vi "TonesLoop_20190705.vi"(7 "WeightOfNewFrequency":dbl=0.1 format="%#_13g", 8 "error in":errorcluster, 11 "Queue in":refnum<queue>) -> (0 "error out":errorcluster)   [LabVIEW 2018]
uses:
  Queue/DataQueueElements.ctl
  Controls/Clusts/ChannelToneData.ctl
  Controls/ToneInfoClust.ctl
  Controls/Clusts/TargetToneData.ctl
  Controls/Clusts/SaturationMonitor.ctl
  Controls/Clusts/Tones_Loop.ctl
  Controls/Clusts/Config_Clust.ctl
  Controls/Clusts/UserConfig.ctl
  Controls/PathsCluster.ctl
  Controls/Clusts/FrontPanel_UserConfig.ctl
  Controls/Clusts/Inclinometer_User_Cfg.ctl
  Controls/Clusts/FP_UserTargetConfig.ctl
  Controls/Clusts/FreqShift.ctl
  Controls/Clusts/FPGA_Scale.ctl
  Controls/Enums/ScaleMeasure.ctl
  Controls/RadioButtons/FilterEnableRadio.ctl
  Controls/Enums/TargetNumber.ctl
  Controls/Clusts/FPGA_Config_Clust.ctl
  Controls/Clusts/NowAllTones.ctl
  Controls/Clusts/FreqFilePaths.ctl
  Controls/Clusts/TonesLogAll.ctl
  Controls/Clusts/ToneLogBuffered.ctl
  Controls/Clusts/SaturationMonitorBuffer.ctl
  Controls/Clusts/AcqData.ctl
  Controls/Clusts/FromFPGA_Clust.ctl
  Controls/Enums/LogLoopEnum.ctl
  Controls/Enums/FP_Loop_Enum.ctl
  Controls/Enums/WatchdogTimer_Enum.ctl
  Controls/Enums/10Hz_Loop_Enum.ctl
  Controls/Clusts/10Hz_Data.ctl
panel:
  in  "1":T1={"Cal"={"Shift_"=-24999462.633451957, "Peak_ToFPGA"=-24999462.633451957, "MaxValue"=0.0, "MaxIndex"=0, "Tone"={"PkLocTrak"=0.0, "PkLocDisp"=0.0, "df_"=0.0, "ZoomPwr"=[], "Phase"=0.0, "PhaseOld"=0.0, "AboveThresh?"=FALSE, "MaxI"=0.0, "MaxQ"=0.0, "median"=0.0, "ISpect"=[], "QSpect"=[], "DeltaPhase"=0.0}, "TimeDomainI"=array[12500 elements], "TimeDomainQ"=array[12500 elements], "PwrSpectrum"=[], "RunningAvgFreq"=0.0, "ISpectPos"=[], "ISpectNeg"=[], "QSpectPos"=[], "QSpectNeg"=[], "10Hz_PwrSpectr"=[], "SNR"=0.0, "AliasWarn"=FALSE, "10Hz_Peak"=[], "ISpect+-"=[], "QSpect+-"=[], "TimeStamp"=timestamp(0 s since 1904-01-01), "I_Index"=array[12500 elements], "Q_Index"=array[12500 elements], "10MHz"=FALSE}, "Beac"={"Shift_"=-24999462.633451957, "Peak_ToFPGA"=-24999462.633451957, "MaxValue"=0.0, "MaxIndex"=0, "Tone"={"PkLocTrak"=0.0, "PkLocDisp"=0.0, "df_"=0.0, "ZoomPwr"=[], "Phase"=0.0, "PhaseOld"=0.0, "AboveThresh?"=FALSE, "MaxI"=0.0, "MaxQ"=0.0, "median"=0.0, "ISpect"=[], "QSpect"=[], "DeltaPhase"=0.0}, "TimeDomainI"=array[12500 elements], "TimeDomainQ"=array[12500 elements], "PwrSpectrum"=[], "RunningAvgFreq"=0.0, "ISpectPos"=[], "ISpectNeg"=[], "QSpectPos"=[], "QSpectNeg"=[], "10Hz_PwrSpectr"=[], "SNR"=0.0, "AliasWarn"=FALSE, "10Hz_Peak"=[], "ISpect+-"=[], "QSpect+-"=[], "TimeStamp"=timestamp(0 s since 1904-01-01), "I_Index"=array[12500 elements], "Q_Index"=array[12500 elements], "10MHz"=FALSE}, "Time"=[], "Saturat"={"MeasMean0"=0.0, "MeasMean1"=0.0, "MeasMax"=0.0, "1_Max"=0.0, "4_Max"=0.0, "5_Max"=0.0, "6_Max"=0.0, "7_Max"=0.0}} {"Beac"."Tone"."median" format="%0.2f"; "Beac"."Tone"."MaxQ" format="%0.2f"; "Cal"."Tone"."median" format="%0.2f"; "Cal"."Tone"."MaxQ" format="%0.2f"}
  in  "Cal":T2={"Shift_"=-24999462.633451957, "Peak_ToFPGA"=-24999462.633451957, "MaxValue"=0.0, "MaxIndex"=0, "Tone"={"PkLocTrak"=0.0, "PkLocDisp"=0.0, "df_"=0.0, "ZoomPwr"=[], "Phase"=0.0, "PhaseOld"=0.0, "AboveThresh?"=FALSE, "MaxI"=0.0, "MaxQ"=0.0, "median"=0.0, "ISpect"=[], "QSpect"=[], "DeltaPhase"=0.0}, "TimeDomainI"=array[12500 elements], "TimeDomainQ"=array[12500 elements], "PwrSpectrum"=[], "RunningAvgFreq"=0.0, "ISpectPos"=[], "ISpectNeg"=[], "QSpectPos"=[], "QSpectNeg"=[], "10Hz_PwrSpectr"=[], "SNR"=0.0, "AliasWarn"=FALSE, "10Hz_Peak"=[], "ISpect+-"=[], "QSpect+-"=[], "TimeStamp"=timestamp(0 s since 1904-01-01), "I_Index"=array[12500 elements], "Q_Index"=array[12500 elements], "10MHz"=FALSE} {"Tone"."median" format="%0.2f"; "Tone"."MaxQ" format="%0.2f"}
  in  "CrossNew":bool
  in  "CoNew":bool
  out "Discard 4":i32
  out "Discard 3":i32
  out "Discard 2":i32
  out "Discard 1":i32
  out "Discard":i32
  out "4 Shift":i32
  out "3 Shift":i32
  out "2 Shift":i32
  out "1 Shift":i32
  out "4 Send":i32
  out "3 Send":i32
  out "2 Send":i32
  out "1 Send":i32
  out "4 Count":i32
  out "3 Count":i32
  out "2 Count":i32
  out "1Count":i32
  out "Tones_Count":i32
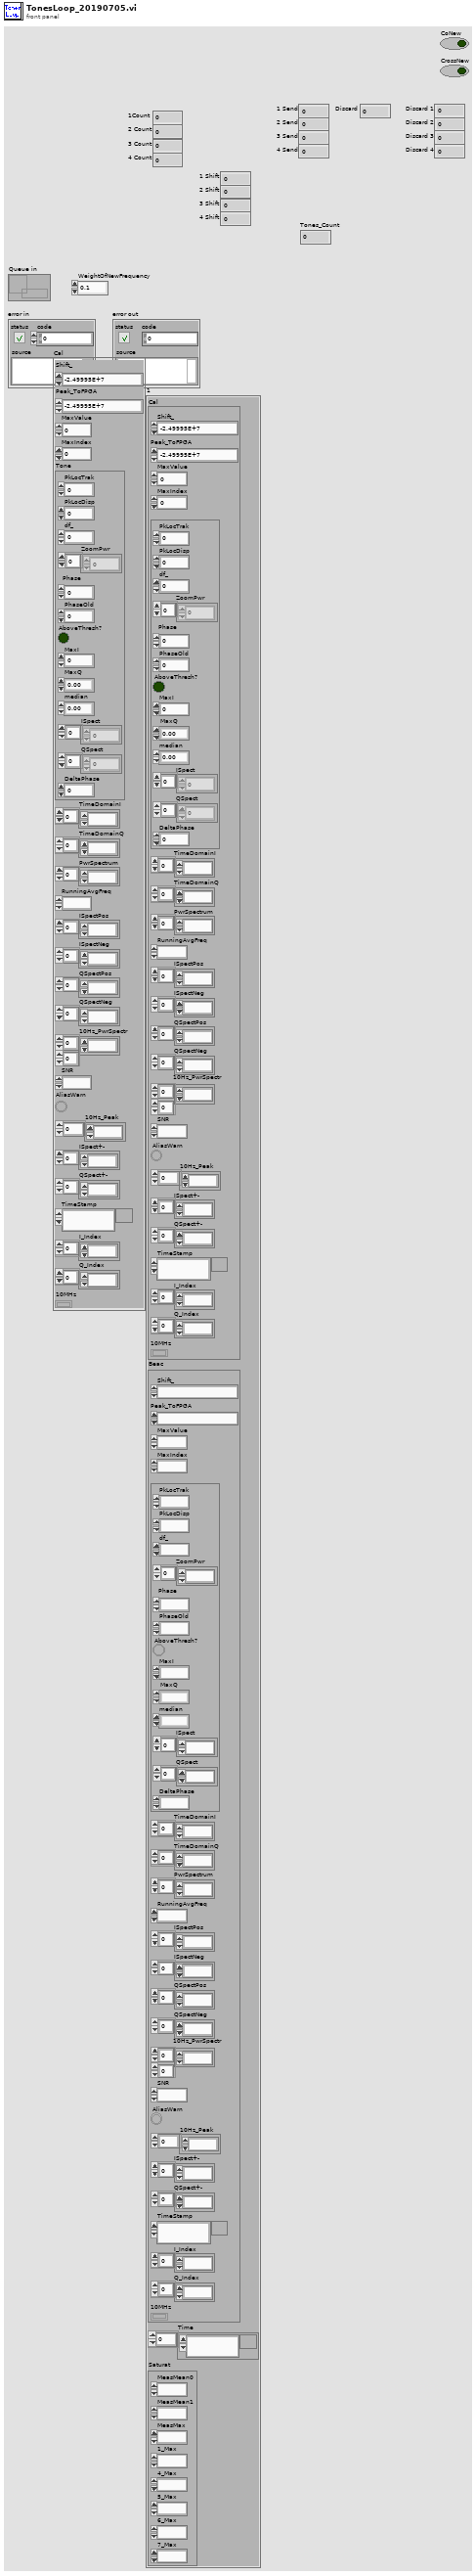
[diagram p1: front panel]
types:
  T1 = typedef "TargetToneData.ctl" = cluster{"Cal":T2, "Beac":T2, "Time":timestamp[], "Saturat":T4}
  T2 = typedef "ChannelToneData.ctl" = cluster{"Shift_":dbl, "Peak_ToFPGA":dbl, "MaxValue":dbl, "MaxIndex":i32, "Tone":T3, "TimeDomainI":ext[], "TimeDomainQ":ext[], "PwrSpectrum":dbl[], "RunningAvgFreq":dbl, "ISpectPos":dbl[], "ISpectNeg":dbl[], "QSpectPos":dbl[], "QSpectNeg":dbl[], "10Hz_PwrSpectr":dbl[][], "SNR":dbl, "AliasWarn":bool, "10Hz_Peak":dbl[], "ISpect+-":dbl[], "QSpect+-":dbl[], "TimeStamp":timestamp, "I_Index":ext[], "Q_Index":ext[], "10MHz":bool}
  T3 = typedef "ToneInfoClust.ctl" = cluster{"PkLocTrak":dbl, "PkLocDisp":dbl, "df_":dbl, "ZoomPwr":dbl[], "Phase":dbl, "PhaseOld":dbl, "AboveThresh?":bool, "MaxI":dbl, "MaxQ":dbl, "median":dbl, "ISpect":dbl[], "QSpect":dbl[], "DeltaPhase":dbl}
  T4 = typedef "SaturationMonitor.ctl" = cluster{"MeasMean0":dbl, "MeasMean1":dbl, "MeasMax":dbl, "1_Max":dbl, "4_Max":dbl, "5_Max":dbl, "6_Max":dbl, "7_Max":dbl}
  T5 = typedef "TonesLogAll.ctl" = cluster{"72co":T6, "72x":T6, "84co":T6, "84x":T6}
  T6 = typedef "ToneLogBuffered.ctl" = cluster{"Count":i32, "CalVal":sgl[], "CalLoc":i32[], "BeacVal":sgl[], "BeacLoc":i32[], "BeacShift":i32[], "Enum":T7, "df":dbl, "PwrSpectr":sgl[][], "ISpectr":sgl[][], "QSpectr":sgl[][], "Time":timestamp[], "SNR":sgl[], "AboveThresh":bool[], "10Hz_PeakVal":dbl[], "Phase":sgl[], "DeltaPhase":dbl[], "Saturat":T8, "10MHz":bool}
  T7 = typedef "TargetNumber.ctl" = enum16{"1", "2", "3", "4"}
  T8 = typedef "SaturationMonitorBuffer.ctl" = cluster{"Meas":bool[], "Stage1":bool[], "Stage4":bool[], "Stage5":bool[], "Stage6":bool[], "Stage7":bool[]}
  T9 = typedef "Tones_Loop.ctl" = cluster{"Config":T10, "FPGA":T20, "Now":T21, "FreqFiles":T22}
  T10 = typedef "Config_Clust.ctl" = cluster{"UsrCfg":T11, "FP_User":T13}
  T11 = typedef "UserConfig.ctl" = cluster{"Paths":T12, "SampleRate":dbl}
  T12 = typedef "PathsCluster.ctl" = cluster{"CfgFile":path, "LogFolder":path, "LogFile":path, "NAS path":path, "ThreshFile":path, "RedunFolder":path}
  T13 = typedef "FrontPanel_UserConfig.ctl" = cluster{"#NoiseSums":u32, "Max_df":u32, "AvgAvg":bool, "#Avg":u16, "AutoCenter":bool, "Inclin":T14, "1":T15, "2":T15, "3":T15, "4":T15, "Target to Probe":T7, "SNR_Thresh":dbl, "Paths":T12, "Connex_Location":string, "SimulateFPGA":bool, "Deadband":dbl}
  T14 = typedef "Inclinometer_User_Cfg.ctl" = cluster{"Vmin":dbl, "Vmax":dbl, "Angle_min":dbl, "Angle_max":dbl, "Offset":dbl, "Pos_Neg":bool}
  T15 = typedef "FP_UserTargetConfig.ctl" = cluster{"Cal_":T16, "Beac":T16, "Scale":T17, "Offset":fxp<+/-,16,16>, "Scale_Noise":fxp<+/-,30,30>, "Scale_Step1":fxp<+/-,17,17>, "Scale_In_RT":ext, "ScaleMeas":fxp<+/-,16,1>, "FreqsToRemove":i32[], "Width":i32[], "ScaleMeasEnum":T18, "FilterEnab":T19}
  T16 = typedef "FreqShift.ctl" = cluster{"Fine":dbl, "Coarse_":dbl}
  T17 = typedef "FPGA_Scale.ctl" = cluster{"Step4":fxp<+/-,23,23>, "Step5":fxp<+/-,23,23>, "Step6":fxp<+/-,23,23>, "Step7":fxp<+/-,23,23>}
  T18 = typedef "ScaleMeasure.ctl" = enum16{"1", "10", "50", "42"}
  T19 = typedef "FilterEnableRadio.ctl" = enum32{"None", "Step 1", "Frequency Shift", "Step 4", "Step 5", "Step 6", "Step 7"}
  T20 = typedef "FPGA_Config_Clust.ctl" = cluster{"Target":T7, "Channel":T7, "Ref1":refnum<k20>, "Ref2":refnum<k20>}
  T21 = typedef "NowAllTones.ctl" = cluster{"Target":T7, "SampleRate":dbl, "AvgFreq":dbl, "72_Shift_":dbl, "84_Shift_":dbl, "1":T1, "2":T1, "3":T1, "4":T1}
  T22 = typedef "FreqFilePaths.ctl" = cluster{"72":path, "84":path}
  T23 = typedef "AcqData.ctl" = cluster{"Data":fxp<+/-,24,1>[], "#":T7, "Saturat":T4, "FromFPGA":T24, "10MHz":bool}
  T24 = typedef "FromFPGA_Clust.ctl" = cluster{"CalTimeDomainI":ext[], "CalTimeDomainI.Index":ext[], "CalTimeDomainQ":ext[], "CalTimeDomainQ.Index":ext[], "BeacTimeDomainI":ext[], "BeacTimeDomainI.Index":ext[], "BeacTimeDomainQ":ext[], "BeacTimeDomainQ.Index":ext[]}
  T25 = typedef "WatchdogTimer_Enum.ctl" = enum16{"ResetAll", "CheckAll", "HW1", "HW2", "Tones", "FP", "Noise", "Log", "TCP", "AI", "TC", "ADAM", "Disdrom", "TE", "Weather"}
  T26 = typedef "FP_Loop_Enum.ctl" = enum16{"FP_Init", "FP_Scale", "FP_Tone", "FP_Noise", "FP_Probes", "FP_PXI", "FP_AI", "FP_TC", "FP_PWR_Hist", "FP_Alarm", "FP_Exit"}
  T27 = typedef "LogLoopEnum.ctl" = enum16{"Log_Init", "Log_Config", "Log_CfgAlarm", "Log_TimeDomain", "Log_Tone", "Log_NoiseTrace", "Log_NoiseSum", "Log_DO", "Log_AI", "Log_TC", "Log_Disdrom", "Log_Weather", "Log_TE", "Log_ADAM", "Log_UPS", "Log_ChkTime", "Log_Alarm", "Log_SSH", "Log_Write", "Log_Exit"}
  T28 = typedef "10Hz_Data.ctl" = cluster{"PeakVal":dbl[], "Channel":T7, "TimeStamp":timestamp}
  T29 = typedef "10Hz_Loop_Enum.ctl" = enum16{"10Hz_Init", "10Hz_Cfg", "10Hz_NewData", "10Hz_Write", "10Hz_Stop"}
  T30 = typedef "DataQueueElements.ctl" = enum16{"Data_Init", "Data_Config", "Data_AddData", "Data_FreqShift", "Data_FPGA_Write", "Data_Transform", "Data_Send", "Data_Exit"}
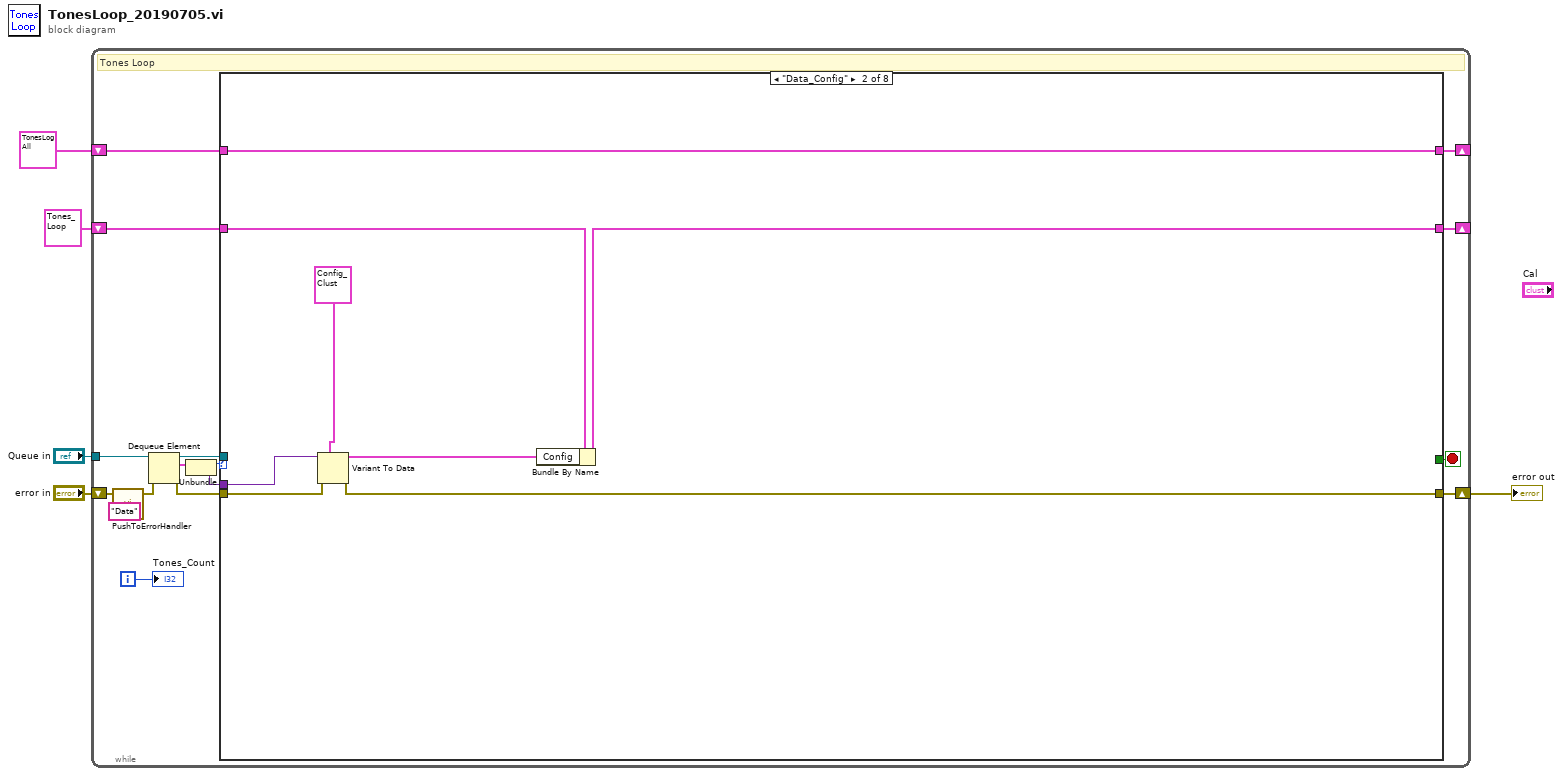
[diagram p0: block diagram]
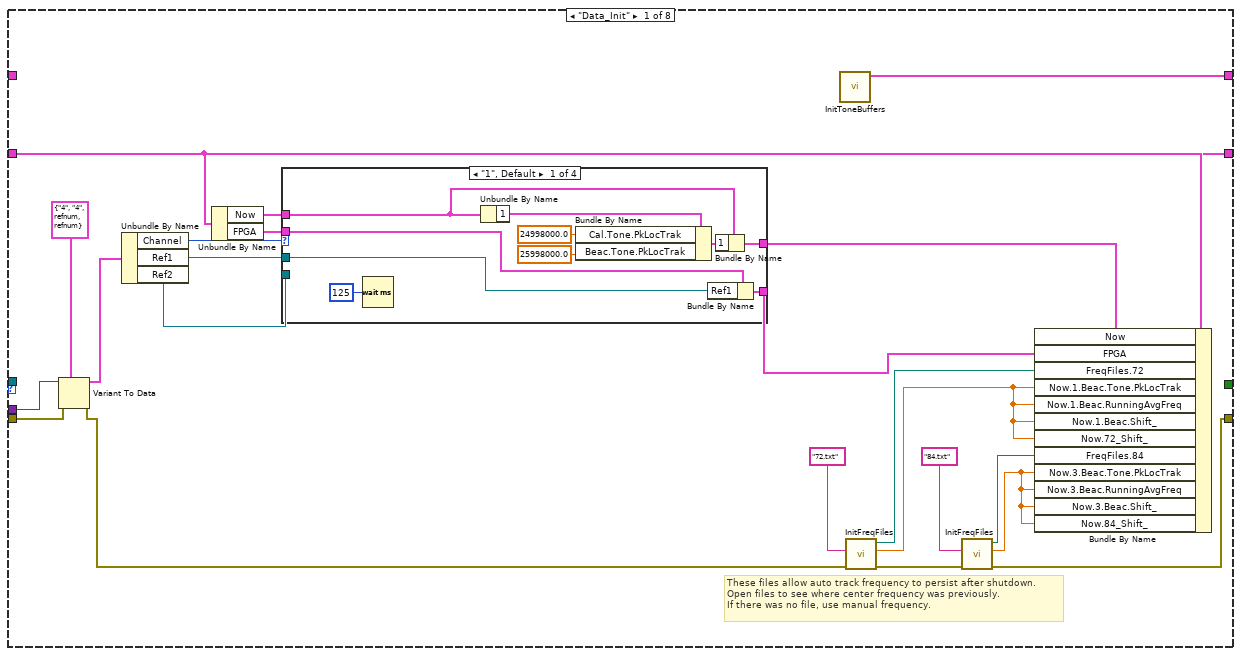
[diagram p2: hidden frame]
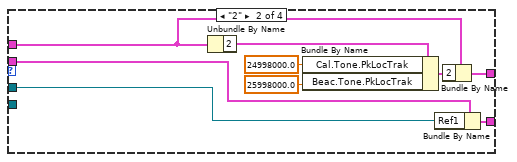
[diagram p3: hidden frame]
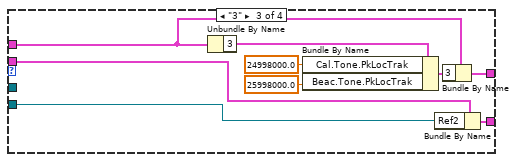
[diagram p4: hidden frame]
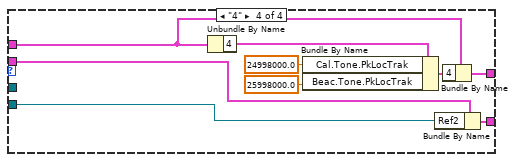
[diagram p5: hidden frame]
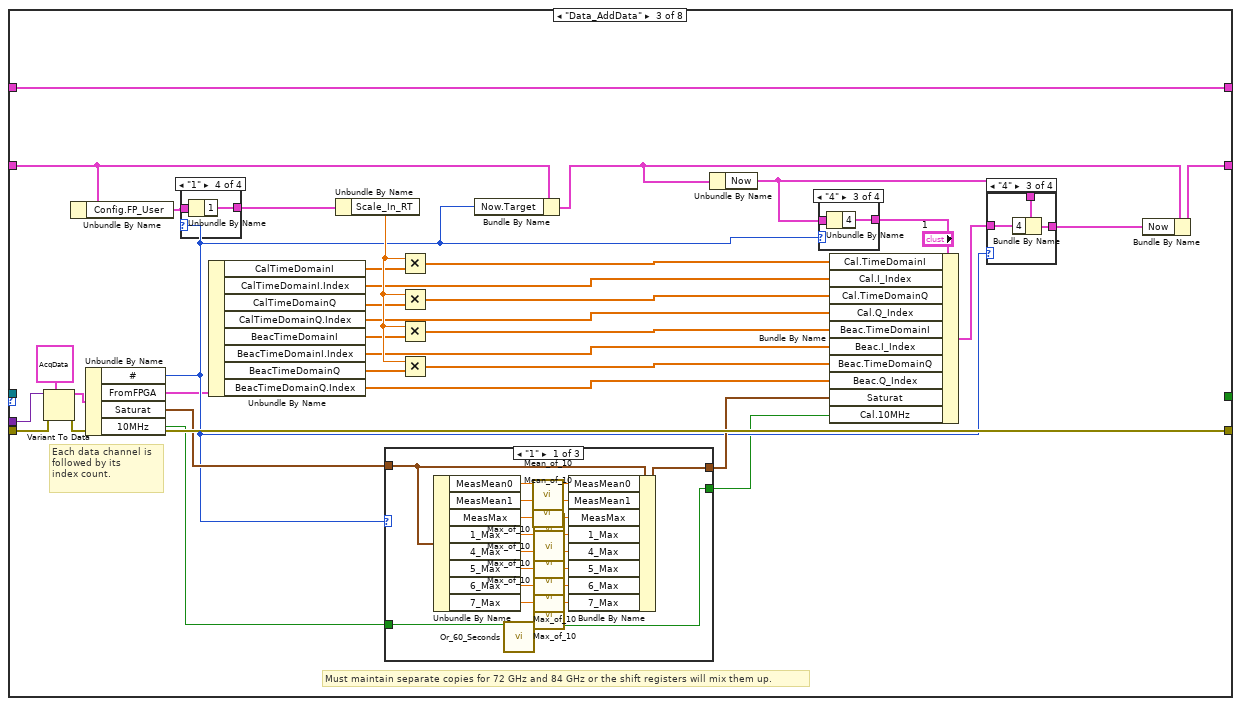
[diagram p6: hidden frame]
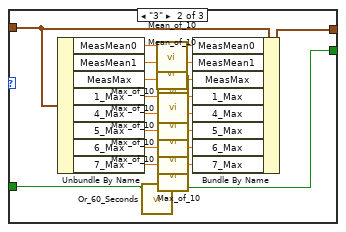
[diagram p7: hidden frame]
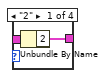
[diagram p9: hidden frame]
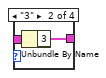
[diagram p10: hidden frame]
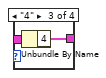
[diagram p11: hidden frame]
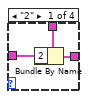
[diagram p12: hidden frame]
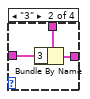
[diagram p13: hidden frame]
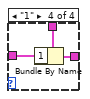
[diagram p14: hidden frame]
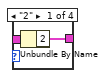
[diagram p15: hidden frame]
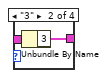
[diagram p16: hidden frame]
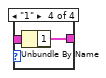
[diagram p17: hidden frame]
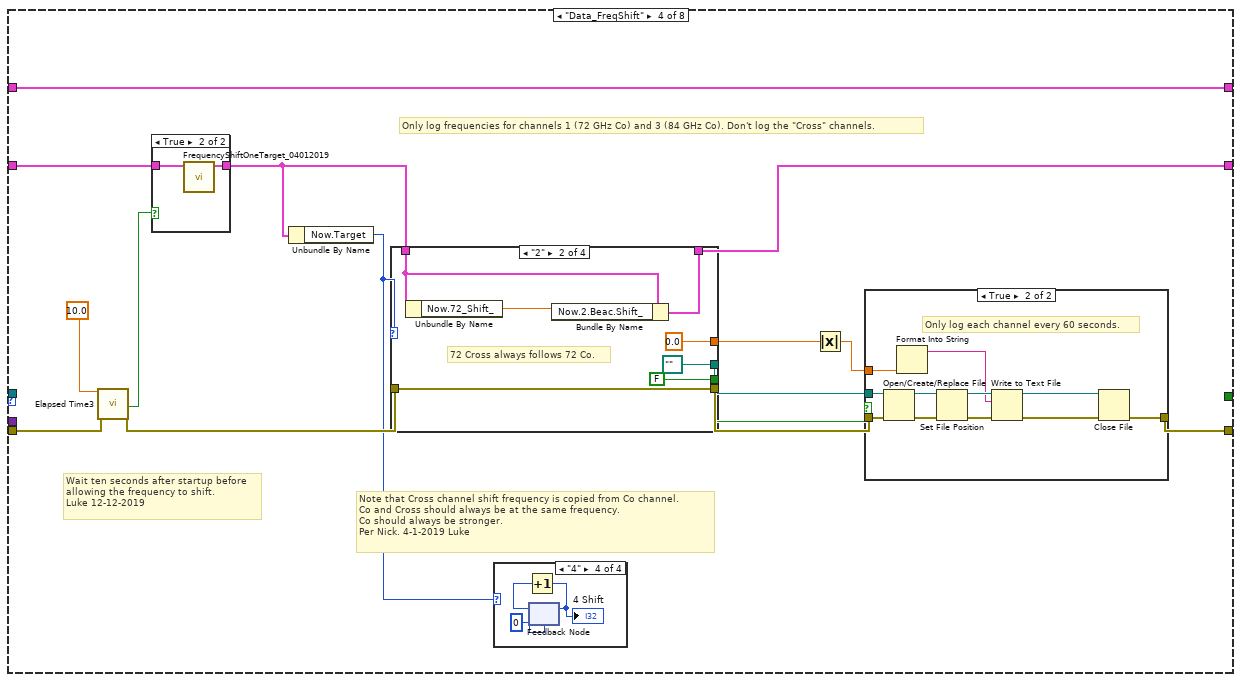
[diagram p18: hidden frame]
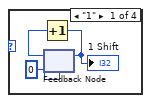
[diagram p19: hidden frame]
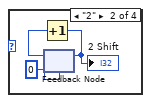
[diagram p20: hidden frame]
diagram:
  n1 = while {
    shift-right: [w14] -> w3
    shift-left: "error in" -> [w19]
    tunnel: "Queue in" -> [w7]
    shift-right: [w11] -> _
    shift-left: T9 {"Config"={"UsrCfg"={"Paths"={"CfgFile"=path "", "LogFolder"=path "", "LogFile"=path "", "NAS path"=path "", "ThreshFile"=path "", "RedunFolder"=path ""}, "SampleRate"=12500.0}, "FP_User"={"#NoiseSums"=1, "Max_df"=1, "AvgAvg"=FALSE, "#Avg"=1, "AutoCenter"=FALSE, "Inclin"={"Vmin"=0.0, "Vmax"=0.0, "Angle_min"=0.0, "Angle_max"=0.0, "Offset"=0.0, "Pos_Neg"=FALSE}, "1"={"Cal_"={"Fine"=0.000213623046875, "Coarse_"=4194303.0}, "Beac"={"Fine"=4194303.0, "Coarse_"=1.0}, "Scale"={"Step4"=10000.0, "Step5"=4194303.0, "Step6"=1.0, "Step7"=10000.0}, "Offset"=0.0, "Scale_Noise"=4194303.0, "Scale_Step1"=65535.0, "Scale_In_RT"=1.0, "ScaleMeas"=0.999969482421875, "FreqsToRemove"=[0, 1633], "Width"=[0, 1633], "ScaleMeasEnum"=enum."50", "FilterEnab"=enum."Step 1"}, "2"={"Cal_"={"Fine"=0.000213623046875, "Coarse_"=4194303.0}, "Beac"={"Fine"=0.000213623046875, "Coarse_"=4194303.0}, "Scale"={"Step4"=0.0, "Step5"=4194303.0, "Step6"=1.0, "Step7"=10000.0}, "Offset"=0.0, "Scale_Noise"=4194303.0, "Scale_Step1"=65535.0, "Scale_In_RT"=1.0, "ScaleMeas"=0.999969482421875, "FreqsToRemove"=[0, 1633], "Width"=[0, 1633], "ScaleMeasEnum"=enum."50", "FilterEnab"=enum."Step 1"}, "3"={"Cal_"={"Fine"=0.000213623046875, "Coarse_"=4194303.0}, "Beac"={"Fine"=0.000213623046875, "Coarse_"=4194303.0}, "Scale"={"Step4"=0.0, "Step5"=4194303.0, "Step6"=1.0, "Step7"=10000.0}, "Offset"=0.0, "Scale_Noise"=4194303.0, "Scale_Step1"=65535.0, "Scale_In_RT"=1.0, "ScaleMeas"=0.999969482421875, "FreqsToRemove"=[0, 1633], "Width"=[0, 1633], "ScaleMeasEnum"=enum."50", "FilterEnab"=enum."Step 1"}, "4"={"Cal_"={"Fine"=0.000213623046875, "Coarse_"=4194303.0}, "Beac"={"Fine"=0.000213623046875, "Coarse_"=4194303.0}, "Scale"={"Step4"=0.0, "Step5"=4194303.0, "Step6"=1.0, "Step7"=10000.0}, "Offset"=0.0, "Scale_Noise"=4194303.0, "Scale_Step1"=1.0, "Scale_In_RT"=10000.0, "ScaleMeas"=0.999969482421875, "FreqsToRemove"=[0, 1633], "Width"=[0, 1633], "ScaleMeasEnum"=enum."50", "FilterEnab"=enum."Step 1"}, "Target to Probe"=enum."4", "SNR_Thresh"=1.0, "Paths"={"CfgFile"=path "", "LogFolder"=path "", "LogFile"=path "", "NAS path"=path "", "ThreshFile"=path "", "RedunFolder"=path ""}, "Connex_Location"="", "SimulateFPGA"=FALSE, "Deadband"=0.0}}, "FPGA"={"Target"=enum."4", "Channel"=enum."4", "Ref1"=refnum, "Ref2"=refnum}, "Now"={"Target"=enum."4", "SampleRate"=0.0, "AvgFreq"=0.0, "72_Shift_"=-24999462.633451957, "84_Shift_"=-24999462.633451957, "1"={"Cal"={"Shift_"=-24999462.633451957, "Peak_ToFPGA"=-24999462.633451957, "MaxValue"=0.0, "MaxIndex"=0, "Tone"={"PkLocTrak"=0.0, "PkLocDisp"=0.0, "df_"=0.0, "ZoomPwr"=[], "Phase"=0.0, "PhaseOld"=0.0, "AboveThresh?"=FALSE, "MaxI"=0.0, "MaxQ"=0.0, "median"=0.0, "ISpect"=[], "QSpect"=[], "DeltaPhase"=0.0}, "TimeDomainI"=array[12500 elements], "TimeDomainQ"=array[12500 elements], "PwrSpectrum"=[], "RunningAvgFreq"=0.0, "ISpectPos"=[], "ISpectNeg"=[], "QSpectPos"=[], "QSpectNeg"=[], "10Hz_PwrSpectr"=[], "SNR"=0.0, "AliasWarn"=FALSE, "10Hz_Peak"=[], "ISpect+-"=[], "QSpect+-"=[], "TimeStamp"=timestamp(0 s since 1904-01-01), "I_Index"=array[12500 elements], "Q_Index"=array[12500 elements], "10MHz"=FALSE}, "Beac"={"Shift_"=-24999462.633451957, "Peak_ToFPGA"=-24999462.633451957, "MaxValue"=0.0, "MaxIndex"=0, "Tone"={"PkLocTrak"=0.0, "PkLocDisp"=0.0, "df_"=0.0, "ZoomPwr"=[], "Phase"=0.0, "PhaseOld"=0.0, "AboveThresh?"=FALSE, "MaxI"=0.0, "MaxQ"=0.0, "median"=0.0, "ISpect"=[], "QSpect"=[], "DeltaPhase"=0.0}, "TimeDomainI"=array[12500 elements], "TimeDomainQ"=array[12500 elements], "PwrSpectrum"=[], "RunningAvgFreq"=0.0, "ISpectPos"=[], "ISpectNeg"=[], "QSpectPos"=[], "QSpectNeg"=[], "10Hz_PwrSpectr"=[], "SNR"=0.0, "AliasWarn"=FALSE, "10Hz_Peak"=[], "ISpect+-"=[], "QSpect+-"=[], "TimeStamp"=timestamp(0 s since 1904-01-01), "I_Index"=array[12500 elements], "Q_Index"=array[12500 elements], "10MHz"=FALSE}, "Time"=[], "Saturat"={"MeasMean0"=0.0, "MeasMean1"=0.0, "MeasMax"=0.0, "1_Max"=0.0, "4_Max"=0.0, "5_Max"=0.0, "6_Max"=0.0, "7_Max"=0.0}}, "2"={"Cal"={"Shift_"=-24999462.633451957, "Peak_ToFPGA"=-24999462.633451957, "MaxValue"=0.0, "MaxIndex"=0, "Tone"={"PkLocTrak"=0.0, "PkLocDisp"=0.0, "df_"=0.0, "ZoomPwr"=[], "Phase"=0.0, "PhaseOld"=0.0, "AboveThresh?"=FALSE, "MaxI"=0.0, "MaxQ"=0.0, "median"=0.0, "ISpect"=[], "QSpect"=[], "DeltaPhase"=0.0}, "TimeDomainI"=array[12500 elements], "TimeDomainQ"=array[12500 elements], "PwrSpectrum"=[], "RunningAvgFreq"=0.0, "ISpectPos"=[], "ISpectNeg"=[], "QSpectPos"=[], "QSpectNeg"=[], "10Hz_PwrSpectr"=[], "SNR"=0.0, "AliasWarn"=FALSE, "10Hz_Peak"=[], "ISpect+-"=[], "QSpect+-"=[], "TimeStamp"=timestamp(0 s since 1904-01-01), "I_Index"=array[12500 elements], "Q_Index"=array[12500 elements], "10MHz"=FALSE}, "Beac"={"Shift_"=-24999462.633451957, "Peak_ToFPGA"=-24999462.633451957, "MaxValue"=0.0, "MaxIndex"=0, "Tone"={"PkLocTrak"=0.0, "PkLocDisp"=0.0, "df_"=0.0, "ZoomPwr"=[], "Phase"=0.0, "PhaseOld"=0.0, "AboveThresh?"=FALSE, "MaxI"=0.0, "MaxQ"=0.0, "median"=0.0, "ISpect"=[], "QSpect"=[], "DeltaPhase"=0.0}, "TimeDomainI"=array[12500 elements], "TimeDomainQ"=array[12500 elements], "PwrSpectrum"=[], "RunningAvgFreq"=0.0, "ISpectPos"=[], "ISpectNeg"=[], "QSpectPos"=[], "QSpectNeg"=[], "10Hz_PwrSpectr"=[], "SNR"=0.0, "AliasWarn"=FALSE, "10Hz_Peak"=[], "ISpect+-"=[], "QSpect+-"=[], "TimeStamp"=timestamp(0 s since 1904-01-01), "I_Index"=array[12500 elements], "Q_Index"=array[12500 elements], "10MHz"=FALSE}, "Time"=[], "Saturat"={"MeasMean0"=0.0, "MeasMean1"=0.0, "MeasMax"=0.0, "1_Max"=0.0, "4_Max"=0.0, "5_Max"=0.0, "6_Max"=0.0, "7_Max"=0.0}}, "3"={"Cal"={"Shift_"=-24999462.633451957, "Peak_ToFPGA"=-24999462.633451957, "MaxValue"=0.0, "MaxIndex"=0, "Tone"={"PkLocTrak"=0.0, "PkLocDisp"=0.0, "df_"=0.0, "ZoomPwr"=[], "Phase"=0.0, "PhaseOld"=0.0, "AboveThresh?"=FALSE, "MaxI"=0.0, "MaxQ"=0.0, "median"=0.0, "ISpect"=[], "QSpect"=[], "DeltaPhase"=0.0}, "TimeDomainI"=array[12500 elements], "TimeDomainQ"=array[12500 elements], "PwrSpectrum"=[], "RunningAvgFreq"=0.0, "ISpectPos"=[], "ISpectNeg"=[], "QSpectPos"=[], "QSpectNeg"=[], "10Hz_PwrSpectr"=[], "SNR"=0.0, "AliasWarn"=FALSE, "10Hz_Peak"=[], "ISpect+-"=[], "QSpect+-"=[], "TimeStamp"=timestamp(0 s since 1904-01-01), "I_Index"=array[12500 elements], "Q_Index"=array[12500 elements], "10MHz"=FALSE}, "Beac"={"Shift_"=-24999462.633451957, "Peak_ToFPGA"=-24999462.633451957, "MaxValue"=0.0, "MaxIndex"=0, "Tone"={"PkLocTrak"=0.0, "PkLocDisp"=0.0, "df_"=0.0, "ZoomPwr"=[], "Phase"=0.0, "PhaseOld"=0.0, "AboveThresh?"=FALSE, "MaxI"=0.0, "MaxQ"=0.0, "median"=0.0, "ISpect"=[], "QSpect"=[], "DeltaPhase"=0.0}, "TimeDomainI"=array[12500 elements], "TimeDomainQ"=array[12500 elements], "PwrSpectrum"=[], "RunningAvgFreq"=0.0, "ISpectPos"=[], "ISpectNeg"=[], "QSpectPos"=[], "QSpectNeg"=[], "10Hz_PwrSpectr"=[], "SNR"=0.0, "AliasWarn"=FALSE, "10Hz_Peak"=[], "ISpect+-"=[], "QSpect+-"=[], "TimeStamp"=timestamp(0 s since 1904-01-01), "I_Index"=array[12500 elements], "Q_Index"=array[12500 elements], "10MHz"=FALSE}, "Time"=[], "Saturat"={"MeasMean0"=0.0, "MeasMean1"=0.0, "MeasMax"=0.0, "1_Max"=0.0, "4_Max"=0.0, "5_Max"=0.0, "6_Max"=0.0, "7_Max"=0.0}}, "4"={"Cal"={"Shift_"=-24999462.633451957, "Peak_ToFPGA"=-24999462.633451957, "MaxValue"=0.0, "MaxIndex"=0, "Tone"={"PkLocTrak"=0.0, "PkLocDisp"=0.0, "df_"=0.0, "ZoomPwr"=[], "Phase"=0.0, "PhaseOld"=0.0, "AboveThresh?"=FALSE, "MaxI"=0.0, "MaxQ"=0.0, "median"=0.0, "ISpect"=[], "QSpect"=[], "DeltaPhase"=0.0}, "TimeDomainI"=array[12500 elements], "TimeDomainQ"=array[12500 elements], "PwrSpectrum"=[], "RunningAvgFreq"=0.0, "ISpectPos"=[], "ISpectNeg"=[], "QSpectPos"=[], "QSpectNeg"=[], "10Hz_PwrSpectr"=[], "SNR"=0.0, "AliasWarn"=FALSE, "10Hz_Peak"=[], "ISpect+-"=[], "QSpect+-"=[], "TimeStamp"=timestamp(0 s since 1904-01-01), "I_Index"=array[12500 elements], "Q_Index"=array[12500 elements], "10MHz"=FALSE}, "Beac"={"Shift_"=-24999462.633451957, "Peak_ToFPGA"=-24999462.633451957, "MaxValue"=0.0, "MaxIndex"=0, "Tone"={"PkLocTrak"=0.0, "PkLocDisp"=0.0, "df_"=0.0, "ZoomPwr"=[], "Phase"=0.0, "PhaseOld"=0.0, "AboveThresh?"=FALSE, "MaxI"=0.0, "MaxQ"=0.0, "median"=0.0, "ISpect"=[], "QSpect"=[], "DeltaPhase"=0.0}, "TimeDomainI"=array[12500 elements], "TimeDomainQ"=array[12500 elements], "PwrSpectrum"=[], "RunningAvgFreq"=0.0, "ISpectPos"=[], "ISpectNeg"=[], "QSpectPos"=[], "QSpectNeg"=[], "10Hz_PwrSpectr"=[], "SNR"=0.0, "AliasWarn"=FALSE, "10Hz_Peak"=[], "ISpect+-"=[], "QSpect+-"=[], "TimeStamp"=timestamp(0 s since 1904-01-01), "I_Index"=array[12500 elements], "Q_Index"=array[12500 elements], "10MHz"=FALSE}, "Time"=[], "Saturat"={"MeasMean0"=0.0, "MeasMean1"=0.0, "MeasMax"=0.0, "1_Max"=0.0, "4_Max"=0.0, "5_Max"=0.0, "6_Max"=0.0, "7_Max"=0.0}}}, "FreqFiles"={"72"=path "", "84"=path ""}} -> [w10]
    shift-right: [w9] -> _
    shift-left: T5 {"72co"={"Count"=0, "CalVal"=[], "CalLoc"=[], "BeacVal"=[], "BeacLoc"=[], "BeacShift"=[], "Enum"=enum."4", "df"=0.0, "PwrSpectr"=[], "ISpectr"=[], "QSpectr"=[], "Time"=[], "SNR"=[], "AboveThresh"=[], "10Hz_PeakVal"=[], "Phase"=[], "DeltaPhase"=[], "Saturat"={"Meas"=[], "Stage1"=[], "Stage4"=[], "Stage5"=[], "Stage6"=[], "Stage7"=[]}, "10MHz"=FALSE}, "72x"={"Count"=0, "CalVal"=[], "CalLoc"=[], "BeacVal"=[], "BeacLoc"=[], "BeacShift"=[], "Enum"=enum."4", "df"=0.0, "PwrSpectr"=[], "ISpectr"=[], "QSpectr"=[], "Time"=[], "SNR"=[], "AboveThresh"=[], "10Hz_PeakVal"=[], "Phase"=[], "DeltaPhase"=[], "Saturat"={"Meas"=[], "Stage1"=[], "Stage4"=[], "Stage5"=[], "Stage6"=[], "Stage7"=[]}, "10MHz"=FALSE}, "84co"={"Count"=0, "CalVal"=[], "CalLoc"=[], "BeacVal"=[], "BeacLoc"=[], "BeacShift"=[], "Enum"=enum."4", "df"=0.0, "PwrSpectr"=[], "ISpectr"=[], "QSpectr"=[], "Time"=[], "SNR"=[], "AboveThresh"=[], "10Hz_PeakVal"=[], "Phase"=[], "DeltaPhase"=[], "Saturat"={"Meas"=[], "Stage1"=[], "Stage4"=[], "Stage5"=[], "Stage6"=[], "Stage7"=[]}, "10MHz"=FALSE}, "84x"={"Count"=0, "CalVal"=[], "CalLoc"=[], "BeacVal"=[], "BeacLoc"=[], "BeacShift"=[], "Enum"=enum."4", "df"=0.0, "PwrSpectr"=[], "ISpectr"=[], "QSpectr"=[], "Time"=[], "SNR"=[], "AboveThresh"=[], "10Hz_PeakVal"=[], "Phase"=[], "DeltaPhase"=[], "Saturat"={"Meas"=[], "Stage1"=[], "Stage4"=[], "Stage5"=[], "Stage6"=[], "Stage7"=[]}, "10MHz"=FALSE}} ("TonesLog") -> [w8]
    i -> [w6]
    stop <- w12 stop-if-true
    # "Tones Loop"
    n2 = call "PushToErrorHandler.vi"("ErrorIn"=w19, "ErrorLocation"="Data") -> ("ErrorOut"=w18:errorcluster)  [unwired: 5 in]
    n3 = Dequeue Element(queue=w7, error in (no error)=w18) -> (queue out=w13:refnum<queue>, element=w21:cluster{"Enum":T30, "Data":variant}, error out=w15:errorcluster)  [unwired: 1 in, 1 out]
    n4 = Unbundle(w21) -> ("Enum"=w20:T30, "Data"=w16:variant)
    n5 = case shown="\"Data_Config\"" w20 {
      tunnel: w16 -> [w44 w85 w123 _ _ _ _ _]
      tunnel: w15 -> [w43 w87 w112 w198 w271 w290 w324 w460]
      tunnel: [w24 w86 w122 w206 w269 w290 w352 w459] -> w14
      tunnel: w13 -> [_ _ _ _ _ _ _ w461]
      tunnel: [_ _ _ _ _ _ _ TRUE] -> w12
      tunnel: [w39 w83 w116 w200 w270 w283 w337 w457] -> w11
      tunnel: w10 -> [w40 w84 w115 w208 w270 w289 w337 w457]
      tunnel: [w31 w82 w111 w207 w268 w275 w340 w456] -> w9
      tunnel: w8 -> [_ w82 w111 w207 w268 w275 w339 w456]
      frame "Data_Init" {
        # "These files allow auto track frequency to persist after shutdown.\nOpen files to see where center frequency was previously.\nIf there was no file, use manual frequency."
        n6 = Variant To Data(error in=w43, type=T20 {"Target"=enum."4", "Channel"=enum."4", "Ref1"=refnum, "Ref2"=refnum} ("FPGA"), Variant=w44) -> (data=w41:T20, error out=w30:errorcluster)
        n7 = Unbundle By Name(w41) -> ("Channel"=w34:T7, "Ref1"=w32:refnum<k20>, "Ref2"=w33:refnum<k20>)
        n8 = Unbundle By Name(w40) -> ("Now"=w38:T21, "FPGA"=w36:T20)
        n9 = case shown="\"1\", Default" w34 {
          tunnel: w38 -> [w50 w59 w68 w77]
          tunnel: [w49 w58 w67 w76] -> w37
          tunnel: w36 -> [w48 w57 w66 w75]
          tunnel: [w47 w56 w65 w74] -> w35
          tunnel: w33 -> [_ _ w64 w73]
          tunnel: w32 -> [w46 w55 _ _]
          frame "1", Default {
            n10 = Wait (ms)(milliseconds to wait=u32 125) -> ()  [unwired: 1 out]
            n11 = Unbundle By Name(w50) -> ("1"=w52:T1)
            n12 = Bundle By Name(cluster=w52, "Cal.Tone.PkLocTrak"=24998000.0 ("Cal.Tone.PeakLoc"), "Beac.Tone.PkLocTrak"=25998000.0 ("Beac.Tone.PeakLoc")) -> (w51:T1)
            n13 = Bundle By Name(cluster=w48, "Ref1"=w46) -> (w47:T20)
            n14 = Bundle By Name(cluster=w50, "1"=w51) -> (w49:T21)
          }
          frame "2" {
            n15 = Unbundle By Name(w59) -> ("2"=w61:T1)
            n16 = Bundle By Name(cluster=w61, "Cal.Tone.PkLocTrak"=24998000.0 ("Cal.Tone.PeakLoc"), "Beac.Tone.PkLocTrak"=25998000.0 ("Beac.Tone.PeakLoc")) -> (w60:T1)
            n17 = Bundle By Name(cluster=w57, "Ref1"=w55) -> (w56:T20)
            n18 = Bundle By Name(cluster=w59, "2"=w60) -> (w58:T21)
          }
          frame "3" {
            n19 = Unbundle By Name(w68) -> ("3"=w70:T1)
            n20 = Bundle By Name(cluster=w70, "Cal.Tone.PkLocTrak"=24998000.0 ("Cal.Tone.PeakLoc"), "Beac.Tone.PkLocTrak"=25998000.0 ("Beac.Tone.PeakLoc")) -> (w69:T1)
            n21 = Bundle By Name(cluster=w66, "Ref2"=w64) -> (w65:T20)
            n22 = Bundle By Name(cluster=w68, "3"=w69) -> (w67:T21)
          }
          frame "4" {
            n23 = Unbundle By Name(w77) -> ("4"=w79:T1)
            n24 = Bundle By Name(cluster=w79, "Cal.Tone.PkLocTrak"=24998000.0 ("Cal.Tone.PeakLoc"), "Beac.Tone.PkLocTrak"=25998000.0 ("Beac.Tone.PeakLoc")) -> (w78:T1)
            n25 = Bundle By Name(cluster=w75, "Ref2"=w73) -> (w74:T20)
            n26 = Bundle By Name(cluster=w77, "4"=w78) -> (w76:T21)
          }
        }
        n27 = call "InitToneBuffers.vi"() -> ("TonesLog"=w31:T5)  [unwired: 11 in]
        n28 = call "InitFreqFiles.vi"("error in"=w30, "FileName"="72.txt") -> ("error out"=w27:errorcluster, "value"=w23:dbl, "path"=w28:path)  [unwired: 7 in]
        n29 = call "InitFreqFiles.vi"("error in"=w27, "FileName"="84.txt") -> ("error out"=w24:errorcluster, "value"=w22:dbl, "path"=w25:path)  [unwired: 7 in]
        n30 = Bundle By Name(cluster=w40, "Now"=w37, "FPGA"=w35, "FreqFiles.72"=w28, "Now.1.Beac.Tone.PkLocTrak"=w23, "Now.1.Beac.RunningAvgFreq"=w23, "Now.1.Beac.Shift_"=w23, "Now.72_Shift_"=w23, "FreqFiles.84"=w25, "Now.3.Beac.Tone.PkLocTrak"=w22, "Now.3.Beac.RunningAvgFreq"=w22, "Now.3.Beac.Shift_"=w22, "Now.84_Shift_"=w22) -> (w39:T9)
      }
      frame "Data_Config" {
        n31 = Variant To Data(error in=w87, type=T10 {"UsrCfg"={"Paths"={"CfgFile"=path "", "LogFolder"=path "", "LogFile"=path "", "NAS path"=path "", "ThreshFile"=path "", "RedunFolder"=path ""}, "SampleRate"=12500.0}, "FP_User"={"#NoiseSums"=1, "Max_df"=1, "AvgAvg"=FALSE, "#Avg"=1, "AutoCenter"=FALSE, "Inclin"={"Vmin"=0.0, "Vmax"=0.0, "Angle_min"=0.0, "Angle_max"=0.0, "Offset"=0.0, "Pos_Neg"=FALSE}, "1"={"Cal_"={"Fine"=0.000213623046875, "Coarse_"=4194303.0}, "Beac"={"Fine"=4194303.0, "Coarse_"=1.0}, "Scale"={"Step4"=10000.0, "Step5"=4194303.0, "Step6"=1.0, "Step7"=10000.0}, "Offset"=0.0, "Scale_Noise"=4194303.0, "Scale_Step1"=65535.0, "Scale_In_RT"=1.0, "ScaleMeas"=0.999969482421875, "FreqsToRemove"=[0, 1633], "Width"=[0, 1633], "ScaleMeasEnum"=enum."50", "FilterEnab"=enum."Step 1"}, "2"={"Cal_"={"Fine"=0.000213623046875, "Coarse_"=4194303.0}, "Beac"={"Fine"=0.000213623046875, "Coarse_"=4194303.0}, "Scale"={"Step4"=0.0, "Step5"=4194303.0, "Step6"=1.0, "Step7"=10000.0}, "Offset"=0.0, "Scale_Noise"=4194303.0, "Scale_Step1"=65535.0, "Scale_In_RT"=1.0, "ScaleMeas"=0.999969482421875, "FreqsToRemove"=[0, 1633], "Width"=[0, 1633], "ScaleMeasEnum"=enum."50", "FilterEnab"=enum."Step 1"}, "3"={"Cal_"={"Fine"=0.000213623046875, "Coarse_"=4194303.0}, "Beac"={"Fine"=0.000213623046875, "Coarse_"=4194303.0}, "Scale"={"Step4"=0.0, "Step5"=4194303.0, "Step6"=1.0, "Step7"=10000.0}, "Offset"=0.0, "Scale_Noise"=4194303.0, "Scale_Step1"=65535.0, "Scale_In_RT"=1.0, "ScaleMeas"=0.999969482421875, "FreqsToRemove"=[0, 1633], "Width"=[0, 1633], "ScaleMeasEnum"=enum."50", "FilterEnab"=enum."Step 1"}, "4"={"Cal_"={"Fine"=0.000213623046875, "Coarse_"=4194303.0}, "Beac"={"Fine"=0.000213623046875, "Coarse_"=4194303.0}, "Scale"={"Step4"=0.0, "Step5"=4194303.0, "Step6"=1.0, "Step7"=10000.0}, "Offset"=0.0, "Scale_Noise"=4194303.0, "Scale_Step1"=1.0, "Scale_In_RT"=10000.0, "ScaleMeas"=0.999969482421875, "FreqsToRemove"=[0, 1633], "Width"=[0, 1633], "ScaleMeasEnum"=enum."50", "FilterEnab"=enum."Step 1"}, "Target to Probe"=enum."4", "SNR_Thresh"=1.0, "Paths"={"CfgFile"=path "", "LogFolder"=path "", "LogFile"=path "", "NAS path"=path "", "ThreshFile"=path "", "RedunFolder"=path ""}, "Connex_Location"="", "SimulateFPGA"=FALSE, "Deadband"=0.0}} ("Config"), Variant=w85) -> (data=w88:T10, error out=w86:errorcluster)
        n32 = Bundle By Name(cluster=w84, "Config"=w88) -> (w83:T9)
      }
      frame "Data_AddData" {
        # "Each data channel is followed by its\nindex count."
        # "Must maintain separate copies for 72 GHz and 84 GHz or the shift registers will mix them up."
        n33 = Variant To Data(error in=w112, type=T23 {"Data"=[], "#"=enum."1", "Saturat"={"MeasMean0"=0.0, "MeasMean1"=0.0, "MeasMax"=0.0, "1_Max"=0.0, "4_Max"=0.0, "5_Max"=0.0, "6_Max"=0.0, "7_Max"=0.0}, "FromFPGA"={"CalTimeDomainI"=[], "CalTimeDomainI.Index"=[], "CalTimeDomainQ"=[], "CalTimeDomainQ.Index"=[], "BeacTimeDomainI"=[], "BeacTimeDomainI.Index"=[], "BeacTimeDomainQ"=[], "BeacTimeDomainQ.Index"=[]}, "10MHz"=FALSE}, Variant=w123) -> (data=w108:T23, error out=w122:errorcluster)
        n34 = Unbundle By Name(w115) -> ("Config.FP_User"=w114:T13)
        n35 = Unbundle By Name(w108) -> ("#"=w105:T7, "FromFPGA"=w104:T24, "Saturat"=w107:T4, "10MHz"=w91:bool)
        n36 = case shown="\"1\"" w105 {
          tunnel: [w167 w169 w171 w173] -> w113
          tunnel: w114 -> [w166 w168 w170 w172]
          frame "2" {
            n37 = Unbundle By Name(w166) -> ("2"=w167:T15)
          }
          frame "3" {
            n38 = Unbundle By Name(w168) -> ("3"=w169:T15)
          }
          frame "4" {
            n39 = Unbundle By Name(w170) -> ("4"=w171:T15)
          }
          frame "1" {
            n40 = Unbundle By Name(w172) -> ("1"=w173:T15)
          }
        }
        n41 = Unbundle By Name(w104) -> ("CalTimeDomainI"=w103:ext[], "CalTimeDomainI.Index"=w98:ext[], "CalTimeDomainQ"=w102:ext[], "CalTimeDomainQ.Index"=w96:ext[], "BeacTimeDomainI"=w101:ext[], "BeacTimeDomainI.Index"=w94:ext[], "BeacTimeDomainQ"=w100:ext[], "BeacTimeDomainQ.Index"=w92:ext[])
        n42 = Unbundle By Name(w113) -> ("Scale_In_RT"=w110:ext)
        n43 = case shown="\"1\"" w105 {
          tunnel: w107 -> [w129 w149 w165]
          tunnel: [w128 w148 w165] -> w106
          tunnel: w91 -> [w125 w145 w164]
          tunnel: [w124 w144 w164] -> w90
          frame "1" {
            n44 = Unbundle By Name(w129) -> ("MeasMean0"=w143:dbl, "MeasMean1"=w141:dbl, "MeasMax"=w127:dbl, "1_Max"=w139:dbl, "4_Max"=w137:dbl, "5_Max"=w136:dbl, "6_Max"=w135:dbl, "7_Max"=w134:dbl)
            n45 = call "Or_60_Seconds.vi"("10MHz?"=w125) -> ("10MHz?_60s"=w124:bool)  [unwired: 9 in, 1 out]
            n46 = call "Mean_of_10.vi"("MeasMean0"=w143) -> ("mean"=w142:dbl)  [unwired: 10 in]
            n47 = call "Mean_of_10.vi"("MeasMean0"=w141) -> ("mean"=w140:dbl)  [unwired: 10 in]
            n48 = call "Max_of_10.vi"("max"=w127) -> ("LongTermMax"=w126:dbl)  [unwired: 10 in]
            n49 = call "Max_of_10.vi"("max"=w139) -> ("LongTermMax"=w138:dbl)  [unwired: 10 in]
            n50 = call "Max_of_10.vi"("max"=w137) -> ("LongTermMax"=w133:dbl)  [unwired: 10 in]
            n51 = call "Max_of_10.vi"("max"=w136) -> ("LongTermMax"=w132:dbl)  [unwired: 10 in]
            n52 = call "Max_of_10.vi"("max"=w135) -> ("LongTermMax"=w131:dbl)  [unwired: 10 in]
            n53 = call "Max_of_10.vi"("max"=w134) -> ("LongTermMax"=w130:dbl)  [unwired: 10 in]
            n54 = Bundle By Name(cluster=w129, "MeasMean0"=w142, "MeasMean1"=w140, "MeasMax"=w126, "1_Max"=w138, "4_Max"=w133, "5_Max"=w132, "6_Max"=w131, "7_Max"=w130) -> (w128:T4)
          }
          frame "3" {
            n55 = Unbundle By Name(w149) -> ("MeasMean0"=w163:dbl, "MeasMean1"=w161:dbl, "MeasMax"=w147:dbl, "1_Max"=w159:dbl, "4_Max"=w157:dbl, "5_Max"=w156:dbl, "6_Max"=w155:dbl, "7_Max"=w154:dbl)
            n56 = call "Or_60_Seconds.vi"("10MHz?"=w145) -> ("10MHz?_60s"=w144:bool)  [unwired: 9 in, 1 out]
            n57 = call "Mean_of_10.vi"("MeasMean0"=w163) -> ("mean"=w162:dbl)  [unwired: 10 in]
            n58 = call "Mean_of_10.vi"("MeasMean0"=w161) -> ("mean"=w160:dbl)  [unwired: 10 in]
            n59 = call "Max_of_10.vi"("max"=w147) -> ("LongTermMax"=w146:dbl)  [unwired: 10 in]
            n60 = call "Max_of_10.vi"("max"=w159) -> ("LongTermMax"=w158:dbl)  [unwired: 10 in]
            n61 = call "Max_of_10.vi"("max"=w157) -> ("LongTermMax"=w153:dbl)  [unwired: 10 in]
            n62 = call "Max_of_10.vi"("max"=w156) -> ("LongTermMax"=w152:dbl)  [unwired: 10 in]
            n63 = call "Max_of_10.vi"("max"=w155) -> ("LongTermMax"=w151:dbl)  [unwired: 10 in]
            n64 = call "Max_of_10.vi"("max"=w154) -> ("LongTermMax"=w150:dbl)  [unwired: 10 in]
            n65 = Bundle By Name(cluster=w149, "MeasMean0"=w162, "MeasMean1"=w160, "MeasMax"=w146, "1_Max"=w158, "4_Max"=w153, "5_Max"=w152, "6_Max"=w151, "7_Max"=w150) -> (w148:T4)
          }
          frame Default {
          }
        }
        n66 = Multiply(x=w110, y=w103) -> (x*y=w99:ext[])
        n67 = Multiply(x=w110, y=w102) -> (x*y=w97:ext[])
        n68 = Multiply(x=w110, y=w101) -> (x*y=w95:ext[])
        n69 = Multiply(x=w110, y=w100) -> (x*y=w93:ext[])
        n70 = Bundle By Name(cluster=w115, "Now.Target"=w105) -> (w109:T9)
        n71 = Unbundle By Name(w109) -> ("Now"=w119:T21)
        n72 = case shown="\"4\"" w105 {
          tunnel: [w187 w189 w191 w193] -> w120
          tunnel: w119 -> [w186 w188 w190 w192]
          frame "2" {
            n73 = Unbundle By Name(w186) -> ("2"=w187:T1)
          }
          frame "3" {
            n74 = Unbundle By Name(w188) -> ("3"=w189:T1)
          }
          frame "4" {
            n75 = Unbundle By Name(w190) -> ("4"=w191:T1)
          }
          frame "1" {
            n76 = Unbundle By Name(w192) -> ("1"=w193:T1)
          }
        }
        n77 = Bundle By Name(cluster=w120, "Cal.TimeDomainI"=w99, "Cal.I_Index"=w98, "Cal.TimeDomainQ"=w97, "Cal.Q_Index"=w96, "Beac.TimeDomainI"=w95, "Beac.I_Index"=w94, "Beac.TimeDomainQ"=w93, "Beac.Q_Index"=w92, "Saturat"=w106, "Cal.10MHz"=w90) -> (w117:T1)
        n78 = case shown="\"4\"" w105 {
          tunnel: w119 -> [w176 w179 w182 w185]
          tunnel: [w175 w178 w181 w184] -> w118
          tunnel: w117 -> [w174 w177 w180 w183]
          frame "2" {
            n79 = Bundle By Name(cluster=w176, "2"=w174) -> (w175:T21)
          }
          frame "3" {
            n80 = Bundle By Name(cluster=w179, "3"=w177) -> (w178:T21)
          }
          frame "4" {
            n81 = Bundle By Name(cluster=w182, "4"=w180) -> (w181:T21)
          }
          frame "1" {
            n82 = Bundle By Name(cluster=w185, "1"=w183) -> (w184:T21)
          }
        }
        n83 = Bundle By Name(cluster=w109, "Now"=w118) -> (w116:T9)
      }
      frame "Data_FreqShift" {
        # "Wait ten seconds after startup before\nallowing the frequency to shift.\nLuke 12-12-2019"
        # "Note that Cross channel shift frequency is copied from Co channel.\nCo and Cross should always be at the same frequency. \nCo should always be stronger.\nPer Nick. 4-1-2019 Luke"
        # "Only log frequencies for channels 1 (72 GHz Co) and 3 (84 GHz Co). Don't log the \"Cross\" channels."
        n84 = call "Elapsed Time3"("Time Target (s)"=10.0, "error in (no error)"=w198) -> ("Time has Elapsed"=w196:bool, "error out"=w199:errorcluster)  [unwired: 10 in, 6 out]
        n85 = case shown="True" w196 {
          tunnel: w208 -> [w221 w223]
          tunnel: [w221 w222] -> w201
          frame False {
          }
          frame True {
            n86 = call "FrequencyShiftOneTarget_04012019.vi"("Tones in"=w223) -> ("Tones out"=w222:T9)  [unwired: 10 in]
          }
        }
        n87 = Unbundle By Name(w201) -> ("Now.Target"=w194:T7)
        n88 = case shown="\"2\"" w194 {
          tunnel: [w232 w236 w248 w252] -> w205
          tunnel: w199 -> [w231 w236 w247 w252]
          tunnel: [w229 FALSE ("Time has Elapsed") w245 FALSE ("Time has Elapsed")] -> w204
          tunnel: [w228 path "" ("72") w244 path "" ("72")] -> w203
          tunnel: [w227 0.0 ("LastPk") w243 0.0 ("LastPk")] -> w202
          tunnel: w201 -> [w226 w234 w242 w250]
          tunnel: [w225 w233 w241 w249] -> w200
          frame "1" {
            n89 = Unbundle By Name(w226) -> ("Now.1.Beac.Shift_"=w224:dbl, "Now.1.Beac.Tone.PkLocTrak"=w227:dbl, "FreqFiles.72"=w228:path)
            n90 = call "Elapsed Time"("Time Target (s)"=60.0, "error in (no error)"=w231) -> ("Time has Elapsed"=w229:bool, "error out"=w232:errorcluster)  [unwired: 10 in, 6 out]
            n91 = Bundle By Name(cluster=w226, "Now.72_Shift_"=w224) -> (w225:T9)
          }
          frame "2" {
            # "72 Cross always follows 72 Co."
            n92 = Unbundle By Name(w234) -> ("Now.72_Shift_"=w235:dbl)
            n93 = Bundle By Name(cluster=w234, "Now.2.Beac.Shift_"=w235) -> (w233:T9)
          }
          frame "3" {
            n94 = Unbundle By Name(w242) -> ("Now.3.Beac.Shift_"=w240:dbl, "Now.3.Beac.Tone.PkLocTrak"=w243:dbl, "FreqFiles.84"=w244:path)
            n95 = call "Elapsed Time2"("Time Target (s)"=60.0, "error in (no error)"=w247) -> ("Time has Elapsed"=w245:bool, "error out"=w248:errorcluster)  [unwired: 10 in, 6 out]
            n96 = Bundle By Name(cluster=w242, "Now.84_Shift_"=w240) -> (w241:T9)
          }
          frame "4" {
            # "72 Cross always follows 72 Co."
            n97 = Unbundle By Name(w250) -> ("Now.84_Shift_"=w251:dbl)
            n98 = Bundle By Name(cluster=w250, "Now.4.Beac.Shift_"=w251) -> (w249:T9)
          }
        }
        n99 = case shown="\"4\"" w194 {
          frame "1" {
            n100 = feedback #1(0) -> (w210:i32)
            n101 = Increment(x=w210) -> (x+1=w211:i32)
            "1 Shift" <- w211
            n102 = feedback-in #1(w211) -> ()
          }
          frame "2" {
            n103 = feedback #2(0) -> (w213:i32)
            n104 = Increment(x=w213) -> (x+1=w214:i32)
            "2 Shift" <- w214
            n105 = feedback-in #2(w214) -> ()
          }
          frame "3" {
            n106 = feedback #3(0) -> (w216:i32)
            n107 = Increment(x=w216) -> (x+1=w217:i32)
            "3 Shift" <- w217
            n108 = feedback-in #3(w217) -> ()
          }
          frame "4" {
            n109 = feedback #4(0) -> (w219:i32)
            n110 = Increment(x=w219) -> (x+1=w220:i32)
            "4 Shift" <- w220
            n111 = feedback-in #4(w220) -> ()
          }
        }
        n112 = Absolute Value(x=w202) -> (abs(x)=w195:dbl)
        n113 = case shown="True" w204 {
          tunnel: [w256 w261] -> w206
          tunnel: w205 -> [w256 w260]
          tunnel: w203 -> [_ w259]
          tunnel: w195 -> [_ w258]
          frame False {
          }
          frame True {
            # "Only log each channel every 60 seconds."
            n114 = Open/Create/Replace File(file path (use dialog)=w259, error in=w260) -> (refnum out=w267:refnum<file>, error out=w264:errorcluster)  [unwired: 4 in, 1 out]
            n115 = Format Into String(w258) -> (resulting string=w257:string)  [unwired: 3 in, 1 out]
            n116 = Set File Position(refnum=w267, error in=w264) -> (refnum out=w266:refnum<file>, error out=w263:errorcluster)  [unwired: 2 in]
            n117 = Write to Text File(file (use dialog)=w266, text=w257, error in=w263) -> (refnum out=w265:refnum<file>, error out=w262:errorcluster)  [unwired: 1 in, 1 out]
            n118 = Close File(refnum=w265, error in=w262) -> (error out=w261:errorcluster)  [unwired: 1 out]
          }
        }
      }
      frame "Data_FPGA_Write" {
        n119 = call "WriteToTarget_20190401.vi"("error in"=w271, "Tones"=w270) -> ("error out"=w269:errorcluster)  [unwired: 9 in]
      }
      frame "Data_Transform" {
        # "Don't need to average.\nNot tracking Cal tone."
        # "Give the system time to stabilize.\nUntil that time, don't use averages,\njust use the newest number."
        # "Perform FFT on both tones from one target (Cal and Beacon from one digitizer)"
        n120 = call "FreqTransformOneChannel.vi"("Tones in"=w289) -> ("Tones out"=w273:T9)  [unwired: 10 in]
        n121 = Unbundle By Name(w273) -> ("Now.Target"=w274:T7)
        n122 = case shown="\"1\"" w274 {
          tunnel: w273 -> [w307 w312 w317 w322]
          tunnel: [w306 w311 w316 w321] -> w286
          tunnel: [w303 w308 w313 w318] -> w280
          frame "1" {
            n123 = Unbundle By Name(w307) -> ("Now.1"=w306:T1)
            n124 = feedback #5(0) -> (w304:i32)
            n125 = Increment(x=w304) -> (x+1=w303:i32)
            "1Count" <- w303
            n126 = feedback-in #5(w303) -> ()
          }
          frame "2" {
            n127 = feedback #6(0) -> (w310:i32)
            n128 = Increment(x=w310) -> (x+1=w308:i32)
            "2 Count" <- w308
            n129 = feedback-in #6(w308) -> ()
            n130 = Unbundle By Name(w312) -> ("Now.2"=w311:T1)
          }
          frame "3" {
            n131 = feedback #7(0) -> (w314:i32)
            n132 = Increment(x=w314) -> (x+1=w313:i32)
            "3 Count" <- w313
            n133 = feedback-in #7(w313) -> ()
            n134 = Unbundle By Name(w317) -> ("Now.3"=w316:T1)
          }
          frame "4" {
            n135 = feedback #8(0) -> (w319:i32)
            n136 = Increment(x=w319) -> (x+1=w318:i32)
            "4 Count" <- w318
            n137 = feedback-in #8(w318) -> ()
            n138 = Unbundle By Name(w322) -> ("Now.4"=w321:T1)
          }
        }
        n139 = Unbundle By Name(w286) -> ("Cal"=w288:T2, "Beac"=w287:T2)
        n140 = Greater?(x=w280, y=100) -> (0:w281:bool)
        n141 = Unbundle By Name(w288) -> ("Tone.PkLocTrak"=w272:dbl)
        n142 = Select(t="WeightOfNewFrequency", s=w281, f=1.0) -> (s? t:f=w276:dbl)
        n143 = Bundle By Name(cluster=w288, "RunningAvgFreq"=w272) -> (w285:T2)
        n144 = call "CalculateRunningAverage.vi"("WeightOfNewFrequency"=w276, "ToneClustIn"=w287) -> ("ToneClustOut"=w284:T2)  [unwired: 6 in, 3 out]
        n145 = Bundle By Name(cluster=w286, "Cal"=w285, "Beac"=w284) -> (w282:T1)
        n146 = case shown="\"2\"" w274 {
          tunnel: w273 -> [w293 w296 w299 w302]
          tunnel: [w292 w295 w298 w301] -> w283
          tunnel: w282 -> [w291 w294 w297 w300]
          frame "1" {
            n147 = Bundle By Name(cluster=w293, "Now.1"=w291) -> (w292:T9)
          }
          frame "2" {
            n148 = Bundle By Name(cluster=w296, "Now.2"=w294) -> (w295:T9)
          }
          frame "3" {
            n149 = Bundle By Name(cluster=w299, "Now.3"=w297) -> (w298:T9)
          }
          frame "4" {
            n150 = Bundle By Name(cluster=w302, "Now.4"=w300) -> (w301:T9)
          }
        }
      }
      frame "Data_Send" {
        w343 = -inf ("number/path/refnum")
        # "Reset\nWatchdog"
        # "Don't log if values are bad."
        # "Send target number with data so it's sorted correctly in the receiving loop."
        n151 = Unbundle By Name(w337) -> ("Now.Target"=w328:T7, "Now"=w338:T21)
        n152 = call "Watchdog_Functional_Global.vi"("Watchdog"=WatchdogTimer_Enum."Tones", "error in"=w324) -> ("error out"=w325:errorcluster)  [unwired: 7 in, 2 out]
        n153 = case shown="\"1\"" w328 {
          selector: w328 -> [w436 w441 w448 w453]
          tunnel: w338 -> [w438 w445 w452 w455]
          tunnel: [w437 w442 w450 w454] -> w345
          tunnel: [w436 w441 w448 w453] -> w336
          tunnel: "CoNew" -> [_ w440 w447 _]
          tunnel: "CrossNew" -> [_ w439 w446 _]
          frame "3" {
            n154 = Unbundle By Name(w438) -> ("3"=w437:T1)
          }
          frame "4" {
            n155 = Unbundle By Name(w445) -> ("3"=w444:T1, "4"=w443:T1)
            n156 = call "CalcDeltaPhase.vi"("CrossNew"=w439, "CoNew"=w440, "Cross"=w443, "Co"=w444) -> ("output cluster"=w442:T1)  [unwired: 7 in]
          }
          frame "2" {
            n157 = Unbundle By Name(w452) -> ("1"=w451:T1, "2"=w449:T1)
            n158 = call "CalcDeltaPhase.vi"("CrossNew"=w446, "CoNew"=w447, "Cross"=w449, "Co"=w451) -> ("output cluster"=w450:T1)  [unwired: 7 in]
          }
          frame "1" {
            n159 = Unbundle By Name(w455) -> ("1"=w454:T1)
          }
        }
        n160 = Unbundle By Name(w345) -> ("Cal.MaxValue"=w344:dbl, "Cal.MaxValue"=w342:dbl)
        n161 = feedback #9(0) -> (w333:i32)
        n162 = case shown="\"1\"" w328 {
          tunnel: [w366 w369] -> w329
          tunnel: w333 -> [w366 _]
          frame Default {
          }
          frame "1" {
            n163 = feedback #10(0) -> (w368:i32)
            n164 = Increment(x=w368) -> (x+1=w369:i32)
            "Discard" <- w369
            n165 = feedback-in #10(w369) -> ()
          }
        }
        n166 = feedback-in #9(w329) -> ()
        n167 = Bundle("Target"=w336, "1"=w345) -> (w350:cluster{"Target":T7, "1":T1})  [unwired: 1 in]
        n168 = To Variant(anything=w350) -> (Variant=w348:variant)
        n169 = Less?(x=w329, y=20) -> (x < y?=w334:bool)
        n170 = Equal?(x=w344, y=w343) -> (x = y?=w335:bool)
        n171 = Equal?(x=w342, y=w343) -> (x = y?=w341:bool)
        n172 = Bundle By Name(cluster=cluster{"Enum":T27, "Data":variant} {"Enum"=enum."Log_Tone", "Data"=variant} ("element"), "Data"=w348) -> (w346:cluster{"Enum":T27, "Data":variant})
        n173 = Bundle By Name(cluster=cluster{"Enum":T26, "Data":variant} {"Enum"=enum."FP_Tone", "Data"=variant}, "Data"=w348) -> (w347:cluster{"Enum":T26, "Data":variant})
        n174 = Compound Arithmetic op=OR(w335, w341, w334) -> (w330:bool)
        n175 = case shown="False" w330 {
          tunnel: [w402 w435] -> w352
          tunnel: w347 -> [w388 _]
          tunnel: w346 -> [w393 _]
          tunnel: w325 -> [w397 w435]
          tunnel: w339 -> [w394 w434]
          tunnel: [w390 w434] -> w340
          tunnel: w336 -> [w373 _]
          tunnel: w337 -> [w371 _]
          frame False {
            # "Send 10 Hz data to Hz log loop"
            # "Send Tone data to FP update loop"
            n176 = Obtain Queue(max queue size (-1, unlimited)=100, name (unnamed)="FP", element data type=w388, error in (no error)=w397) -> (queue out=w401:refnum<queue>, error out=w400:errorcluster)  [unwired: 1 in, 1 out]
            n177 = Unbundle By Name(w371) -> ()  [unwired: 1 out]
            n178 = Enqueue Element(queue=w401, element=w388, timeout in ms (-1)=10, error in (no error)=w400) -> (queue out=w396:refnum<queue>, error out=w395:errorcluster)  [unwired: 1 out]
            n179 = Release Queue(queue=w396, error in (no error)=w395) -> (error out=w381:errorcluster)  [unwired: 1 in, 2 out]
            n180 = call "SortToneDataForLogging.vi"("Target"=w373, "element in"=w393, "TonesLog"=w394) -> ("SendToQueue"=w392:cluster{"Enum":T27, "Data":variant}, "Full set"=w391:bool, "TonesLog w/ New Data"=w390:T5, "Target"=w370:T7, "10Hz_Time"=w372:timestamp, "10Hz_PeakVal"=w374:dbl[])  [unwired: 3 in]
            n181 = Bundle By Name(cluster=T28 {"PeakVal"=[], "Channel"=enum."4", "TimeStamp"=timestamp(0 s since 1904-01-01)} ("Data"), "TimeStamp"=w372, "Channel"=w370, "PeakVal"=w374) -> (w376:T28)
            n182 = case shown="\"1\"" w370 {
              frame "1" {
                n183 = feedback #11(0) -> (w404:i32)
                n184 = Increment(x=w404) -> (x+1=w405:i32)
                "1 Send" <- w405
                n185 = feedback-in #11(w405) -> ()
              }
              frame "2" {
                n186 = feedback #12(0) -> (w407:i32)
                n187 = Increment(x=w407) -> (x+1=w408:i32)
                "2 Send" <- w408
                n188 = feedback-in #12(w408) -> ()
              }
              frame "3" {
                n189 = feedback #13(0) -> (w410:i32)
                n190 = Increment(x=w410) -> (x+1=w411:i32)
                "3 Send" <- w411
                n191 = feedback-in #13(w411) -> ()
              }
              frame "4" {
                n192 = feedback #14(0) -> (w413:i32)
                n193 = Increment(x=w413) -> (x+1=w414:i32)
                "4 Send" <- w414
                n194 = feedback-in #14(w414) -> ()
              }
            }
            n195 = To Variant(anything=w376) -> (Variant=w375:variant)
            n196 = Bundle By Name(cluster=cluster{"Enum":T29, "Var":variant} {"Enum"=enum."10Hz_NewData", "Var"=variant}, "Var"=w375) -> (w379:cluster{"Enum":T29, "Var":variant})
            n197 = Obtain Queue(max queue size (-1, unlimited)=100, name (unnamed)="10Hz", element data type=w379, error in (no error)=w381) -> (queue out=w385:refnum<queue>, error out=w386:errorcluster)  [unwired: 1 in, 1 out]
            n198 = case shown="\"1\", \"3\"" w370 {
              tunnel: w386 -> [w415 w422]
              tunnel: w385 -> [w416 w421]
              tunnel: [w415 w420] -> w382
              tunnel: w379 -> [_ w419]
              tunnel: [w416 w418] -> w378
              frame Default {
              }
              frame "1", "3" {
                n199 = Enqueue Element(queue=w421, element=w419, timeout in ms (-1)=10, error in (no error)=w422) -> (queue out=w418:refnum<queue>, error out=w420:errorcluster)  [unwired: 1 out]
              }
            }
            n200 = Release Queue(queue=w378, error in (no error)=w382) -> (error out=w387:errorcluster)  [unwired: 1 in, 2 out]
            n201 = case shown="True" w391 {
              tunnel: [w423 w433] -> w402
              tunnel: w387 -> [w423 w432]
              tunnel: w392 -> [_ w425]
              frame False {
              }
              frame True {
                # "Send Tone data to Log loop"
                n202 = Obtain Queue(max queue size (-1, unlimited)=100, name (unnamed)="Log", element data type=w425, error in (no error)=w432) -> (queue out=w428:refnum<queue>, error out=w429:errorcluster)  [unwired: 1 in, 1 out]
                n203 = Enqueue Element(queue=w428, element=w425, timeout in ms (-1)=10, error in (no error)=w429) -> (queue out=w426:refnum<queue>, error out=w427:errorcluster)  [unwired: 1 out]
                n204 = Release Queue(queue=w426, error in (no error)=w427) -> (error out=w433:errorcluster)  [unwired: 1 in, 2 out]
              }
            }
          }
          frame True {
          }
        }
        n205 = case shown="True" w330 {
          tunnel: w328 -> [_ w353]
          frame False {
          }
          frame True {
            n206 = case shown="\"2\"" w353 {
              tunnel: [w356 w359 w362 w365] -> _
              frame "1" {
                n207 = feedback #15(0) -> (w355:i32)
                n208 = Increment(x=w355) -> (x+1=w356:i32)
                "Discard 1" <- w356
                n209 = feedback-in #15(w356) -> ()
              }
              frame "2" {
                n210 = feedback #16(0) -> (w358:i32)
                n211 = Increment(x=w358) -> (x+1=w359:i32)
                "Discard 2" <- w359
                n212 = feedback-in #16(w359) -> ()
              }
              frame "3" {
                n213 = feedback #17(0) -> (w361:i32)
                n214 = Increment(x=w361) -> (x+1=w362:i32)
                "Discard 3" <- w362
                n215 = feedback-in #17(w362) -> ()
              }
              frame "4" {
                n216 = feedback #18(0) -> (w364:i32)
                n217 = Increment(x=w364) -> (x+1=w365:i32)
                "Discard 4" <- w365
                n218 = feedback-in #18(w365) -> ()
              }
            }
          }
        }
      }
      frame "Data_Exit" {
        # "This case is called upon program exit and will close this queue and exit the loop"
        n219 = Release Queue(queue=w461, error in (no error)=w460) -> (error out=w459:errorcluster)  [unwired: 1 in, 2 out]
      }
    }
    "Tones_Count" <- w6
  }
  "error out" <- w3
